vi "formge.vi"(7 "base path":path=path "D:/control", 9 "Message Data":string[][](array[string]), 10 "Message":string[](array[string])) -> ()   [LabVIEW 2015]
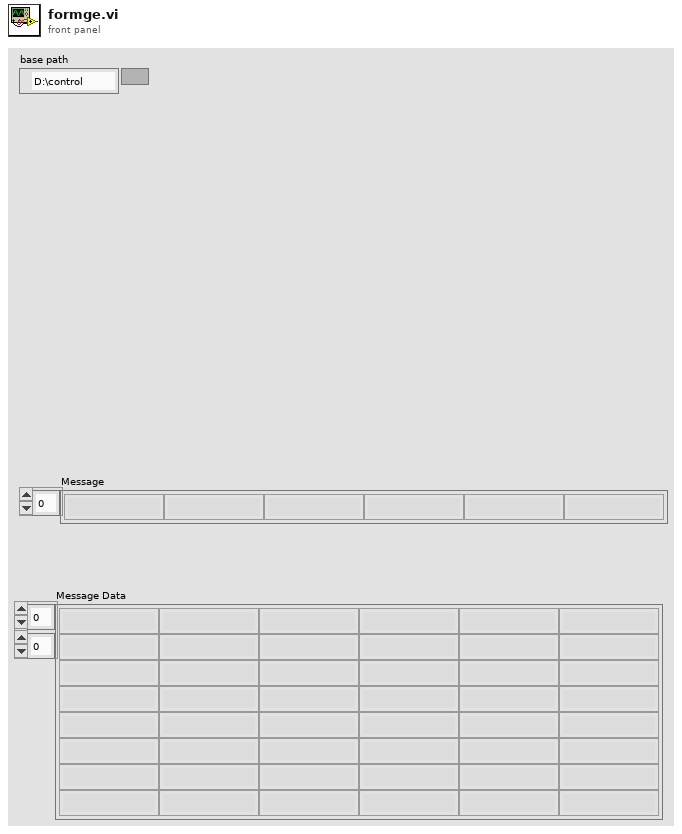
[diagram p1: front panel]
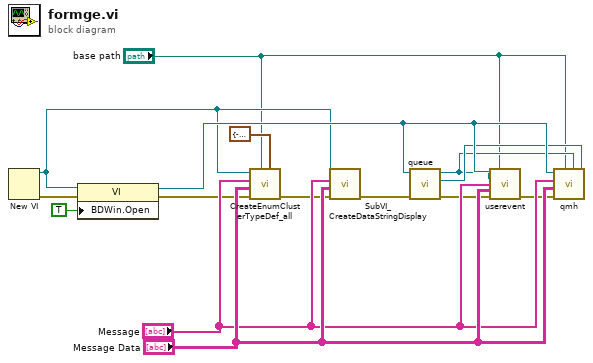
[diagram p0: block diagram]
diagram:
  n1 = New VI() -> (0:w14:errorcluster, 3:w8:refnum<vi>)  [unwired: 7 in]
  n2 = property class="VI"(reference=w8, error in=w14, "BDWin.Open"=TRUE ("Block Diagram Window:Open")) -> (reference out=w12:refnum<vi>, error out=w9:errorcluster)
  n3 = call "CreateEnumClusterTypeDef_all.vi"("BP_Point(0,0)"=cluster{"Width":i32, "Height":i32} {"Width"=-65, "Height"=0}, "base path"="base path", "error in (no error)"=w9, "Data"="Message Data", "DataName"="Message", "VI in"=w8) -> ("error out"=w7:errorcluster)  [unwired: 4 in, 1 out]
  n4 = call "SubVI_CreateDataStringDisplay.vi"("error in (no error)"=w7, "Data"="Message Data", "DataName"="Message", "VI in"=w8) -> ("error out"=w4:errorcluster)  [unwired: 6 in, 1 out]
  n5 = call "queue.vi"("error in (no error)"=w4, "VI in"=w12) -> ("error out"=w5:errorcluster, "queueErrorTerm"=w3:refnum<vi>, "Terminal out"=w2:refnum<vi>)  [unwired: 7 in]
  n6 = call "userevent.vi"("VI in"=w12, "Path"="base path", "Queue in"=w2, "DataName"="Message", "Data"="Message Data", "error in (no error)"=w5) -> ("error out"=w6:errorcluster)  [unwired: 9 in]
  n7 = call "qmh.vi"("errorTerm in"=w3, "Terminal In"=w2, "base path"="base path", "error in (no error)"=w6, "Data"="Message Data", "DataName"="Message", "VI in"=w12) -> ()  [unwired: 4 in, 1 out]
